vi "Example Callback.vi"() -> ()   [LabVIEW 2013]
uses:
  C:/tf/play/labview/Tinkerforge.dll
  Tinkerforge.dll
panel:
  in  "stop":bool
  out "temperature (°C)":sgl format="%#_13g"
  in  "uid":string="amb"
  in  "port":i32=4223
  in  "host":string="localhost"
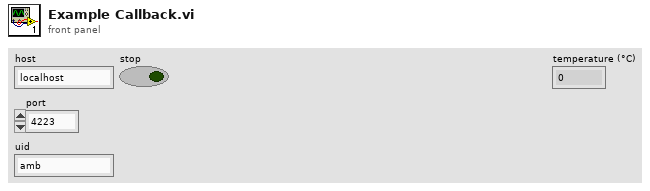
[diagram p1: front panel]
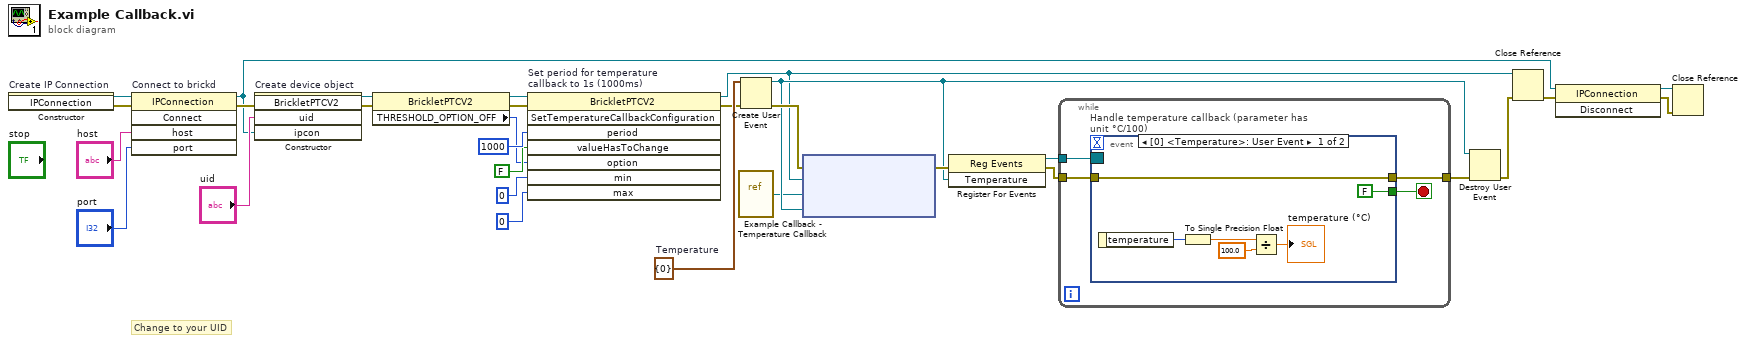
[diagram p0: block diagram]
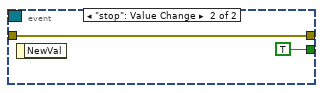
[diagram p2: hidden frame]
diagram:
  w14 = cluster{"temperature":i32} {"temperature"=0}  # Temperature
  # "Change to your UID"
  n1 = constructor on="Create IP Connection" class="IPConnection"() -> (reference out=w30:refnum<k24>, error out=w10:errorcluster)  [unwired: 3 in, 1 out]
  n2 = invoke on="Connect to brickd" class="IPConnection" method="Connect"(reference=w30, error in=w10, "host"="host", "port"="port") -> (reference out=w23:refnum<k24>, error out=w26:errorcluster)  [unwired: 1 in, 3 out]
  n3 = constructor on="Create device object" class="BrickletPTCV2"(error in=w26, "uid"="uid", "ipcon"=w23) -> (reference out=w3:refnum<k24>, error out=w5:errorcluster)  [unwired: 2 in, 3 out]
  n4 = property class="BrickletPTCV2"(reference=w3, error in=w5) -> (reference out=w2:refnum<k24>, error out=w4:errorcluster, "THRESHOLD_OPTION_OFF"=w1:u16)
  n5 = invoke on="Set period for temperature\ncallback to 1s (1000ms)" class="BrickletPTCV2" method="SetTemperatureCallbackConfiguration"(reference=w2, error in=w4, "period"=i64 1000, "valueHasToChange"=FALSE, "option"=w1, "min"=0, "max"=0) -> (reference out=w12:refnum<k24>, error out=w13:errorcluster)  [unwired: 1 in, 6 out]
  n6 = vi-ref "Example Callback - Temperature Callback.vi"() -> ("vi reference"=w9:refnum<vi>)
  n7 = Create User Event(user event datatype=w14, error in=w13) -> (user event=w16:refnum<user-event>, error out=w21:errorcluster)
  n8 = node ("Register Event Callback")(w21, w12, w9, w16) -> (w20:errorcluster)  [unwired: 1 in, 1 out]
  n9 = register-events(error in=w20, w16) -> (reference out=w19:refnum<event-registration>, error out=w17:errorcluster)  [unwired: 1 in]
  n10 = while {
    tunnel: w19 -> [w34]
    tunnel: [w33] -> w18
    tunnel: w17 -> [w32]
    stop <- w31 stop-if-true
    n11 = event "Handle temperature callback (parameter has unit °C/100)" shown="[0] <Temperature>: User Event" {
      selector: w34 -> [_ _]
      dyn-events: _ -> [_ _]
      timeout: _ -> [_ _]
      tunnel: [w37 w41] -> w33
      tunnel: w32 -> [w37 w41]
      tunnel: [FALSE TRUE] -> w31
      event User Event {
        n12 = event-data() -> ("temperature"=w38:i32)  [unwired: 1 in]
        n13 = To Single Precision Float(number=w38) -> (single precision float=w39:sgl)
        n14 = Divide(x=w39, y=sgl 100.0) -> (x/y=→"temperature (°C)":sgl)
      }
      event "stop": Value Change {
        n15 = event-data() -> ()  [unwired: 1 in, 1 out]
      }
    }
  }
  n16 = Destroy User Event(user event=w16, error in=w18) -> (error out=w15:errorcluster)
  n17 = Close Reference(reference=w12, error in (no error)=w15) -> (error out=w25:errorcluster)
  n18 = invoke class="IPConnection" method="Disconnect"(reference=w23, error in=w25) -> (reference out=w22:refnum<k24>, error out=w24:errorcluster)  [unwired: 1 in, 1 out]
  n19 = Close Reference(reference=w22, error in (no error)=w24) -> ()  [unwired: 1 out]
